vi "SetAmp.vi"(2 "error in":errorcluster, 3 "Amplitude":i32=44, 4 "Supply":enum16{"Negative", "Positive"}(ring), 5 "Daxsonics FTDI controller":refnum<visa-resource-name>) -> (0 "error out":errorcluster, 1 "VISA resource name out":refnum<visa-resource-name>)   [LabVIEW 2022 SP3]
uses:
  <vilib>/Instr/_visa.llb/VISA Configure Serial Port (Instr).vi
panel:
  out "Command String":string
  out "read buffer":string
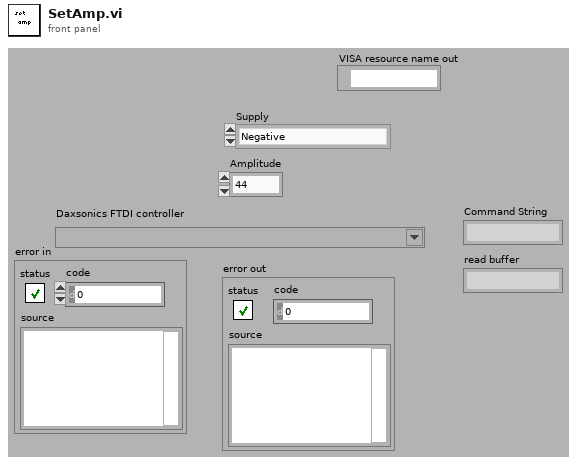
[diagram p1: front panel]
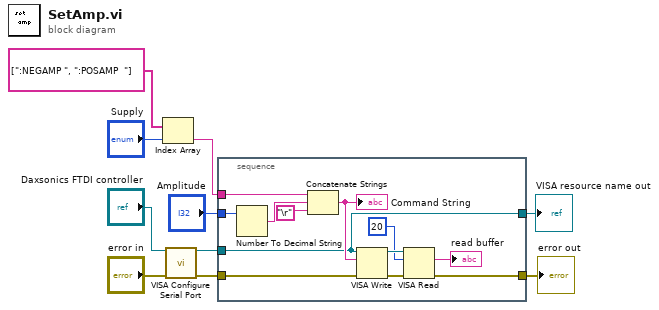
[diagram p0: block diagram]
diagram:
  n1 = Index Array(array=string[] [":NEGAMP ", ":POSAMP  "], index="Supply") -> (element=w3:string)
  n2 = call-poly "VISA Configure Serial Port"("VISA resource name"="Daxsonics FTDI controller", "error in (no error)"="error in") -> ("VISA resource name out"=w9:refnum<visa-resource-name>, "error out"=w8:errorcluster)  [unwired: 12 in]
  n3 = stacked-sequence {
    tunnel: [w12] -> w1
    tunnel: "Amplitude" -> [w22]
    tunnel: w8 -> [w21]
    tunnel: [w13] -> w7
    tunnel: w9 -> [w12]
    tunnel: w3 -> [w11]
    frame #0 {
      n4 = Number To Decimal String(number=w22) -> (decimal integer string=w20:string)  [unwired: 1 in]
      n5 = Concatenate Strings(w11, w20, "\r") -> (w19:string)
      "Command String" <- w19
      n6 = VISA Write(VISA resource name=w12, write buffer=w19, error in (no error)=w21) -> (VISA resource name out=w17:refnum<visa-resource-name>, error out=w16:errorcluster)  [unwired: 1 out]
      n7 = VISA Read(VISA resource name=w17, byte count=u32 20, error in (no error)=w16) -> (read buffer=→"read buffer":string, error out=w13:errorcluster)  [unwired: 2 out]
    }
  }
  "error out" <- w7
  "VISA resource name out" <- w1
